vi "VI Server_TREE_ClearSymbols_and_Backgrounds.vi"(7 "Label":string, 8 "error in":errorcluster, 9 "Tree.Ref":refnum<vi>, 11 "VI Server.RefsCluster":T1) -> (0 "error out":errorcluster, 1 "Tree.Ref.DUP":refnum<vi>, 3 "VI Server.RefsCluster.DUP":T1)   [LabVIEW 2020]
uses:
  VI Server_TypeDefs/VI Server_RefsCluster.ctl
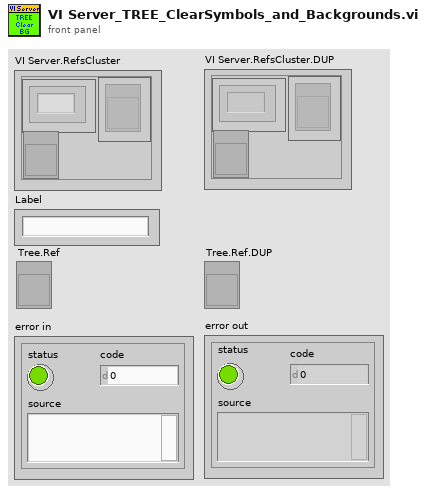
[diagram p1: front panel]
types:
  T1 = typedef "VI Server_RefsCluster.ctl" = cluster{"Labels":string[], "Refs":refnum<vi>[], "VI Ref":refnum<vi>}
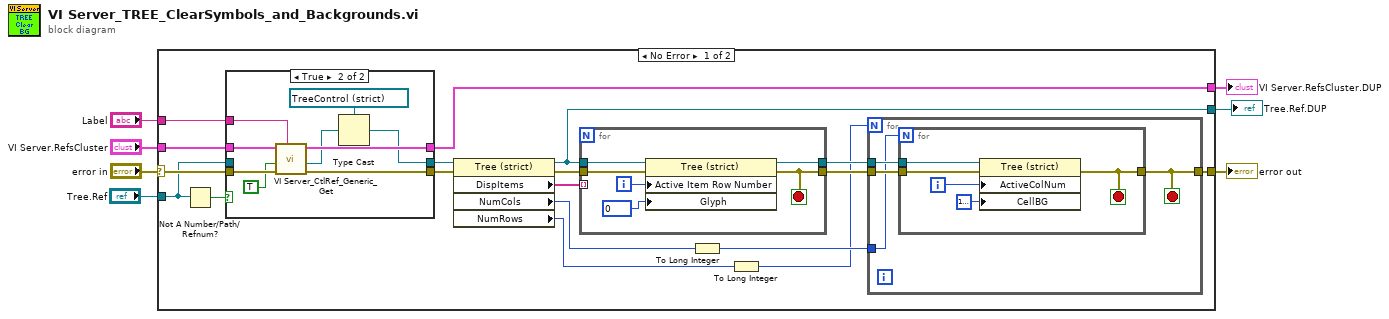
[diagram p0: block diagram]
diagram:
  n1 = case shown="No Error" "error in" {
    selector: "error in" -> [w25 w54]
    tunnel: [w13 w54] -> w6
    tunnel: "VI Server.RefsCluster" -> [w24 w53]
    tunnel: [w23 w53] -> w4
    tunnel: "Label" -> [w22 _]
    tunnel: [w17 _] -> w1
    tunnel: "Tree.Ref" -> [w20 _]
    frame No Error {
      n2 = Not A Number/Path/Refnum?(number/path/refnum=w20) -> (NaN/Path/Refnum?=w21:bool)
      n3 = case shown="True" w21 {
        tunnel: w25 -> [w43 w52]
        tunnel: w24 -> [w41 w51]
        tunnel: [w41 w50] -> w23
        tunnel: w22 -> [_ w49]
        tunnel: [w42 w47] -> w18
        tunnel: [w43 w46] -> w19
        tunnel: w20 -> [w42 _]
        frame False {
        }
        frame True {
          n4 = call "VI Server_CtlRef_Generic_Get.vi"("Control.Label"=w49, "error in"=w52, "SingleInstance"=TRUE, "VI Server.RefsCluster"=w51) -> ("error out"=w46:errorcluster, "Control.Ref.Generic"=w48:refnum<vi>, "VI Server.RefsCluster.DUP"=w50:T1)  [unwired: 5 in]
          n5 = Type Cast(type=refnum<vi> refnum ("Test.Tree"), x=w48) -> (*(type *) &x=w47:refnum<vi>)
        }
      }
      n6 = property class="Tree (strict)"(reference=w18, error in=w19) -> (reference out=w17:refnum<vi>, error out=w16:errorcluster, "DispItems"=w15:string[], "NumCols"=w11:u32, "NumRows"=w9:u32)
      n7 = for {
        tunnel: w17 -> [w39]
        tunnel: w15 -> [_] mode=indexing
        tunnel: w16 -> [w38]
        tunnel: [w36] -> w14
        tunnel: [w35] -> w12
        i -> [w37]
        stop <- w36 stop-if-true
        n8 = property on="Property Node" class="Tree (strict)"(reference=w39, error in=w38, "Active Item Row Number"=w37, "Glyph"=0) -> (reference out=w35:refnum<vi>, error out=w36:errorcluster)
      }
      n9 = To Long Integer(number=w11) -> (32bit integer=w10:i32)
      n10 = To Long Integer(number=w9) -> (32bit integer=w8:i32)
      n11 = for {
        N: w8 -> [_]
        tunnel: w12 -> [w28]
        tunnel: w10 -> [w27]
        tunnel: w14 -> [w29]
        tunnel: [w26] -> w13
        stop <- w26 stop-if-true
        n12 = for {
          N: w27 -> [_]
          tunnel: w29 -> [w34]
          tunnel: [w33] -> w26
          tunnel: w28 -> [w30]
          i -> [w32]
          stop <- w33 stop-if-true
          n13 = property on="Property Node" class="Tree (strict)"(reference=w30, error in=w34, "ActiveColNum"=w32, "CellBG"=u32 16777226) -> (error out=w33:errorcluster)  [unwired: 1 out]
        }
      }
    }
    frame Error {
    }
  }
  "VI Server.RefsCluster.DUP" <- w4
  "error out" <- w6
  "Tree.Ref.DUP" <- w1
